vi "Convert Write ERD List to Message.vi"(0 "GEA Inputs":T1 {"Destination" format="%.0x"; "Source" format="%.0x"}, 7 "Write ERD List":T3[](array[typedef]) {"ERD Number" format="%.0x"}, 11 "Error In":errorcluster) -> (4 "GEA Message":T2 {"Command" format="%02x"; "Destination" format="%02x"; "Source" format="%02x"}, 15 "Error Out":errorcluster)   [LabVIEW 2016, in "GEA2_Toolkit.lvlib"]
doc: "This vi uses the Source / Destination from the GEA input and the ERD Write list to format a single GEA2 message to read the list of ERDs."
uses:
  library/GEA2_Toolkit.lvlib
  type defs/ERD Write Data In.ctl
  type defs/Data Type.ctl
  type defs/Data In.ctl
  type defs/Source_Destination.ctl
  <vilib>/regexp/Match Regular Expression.xnode
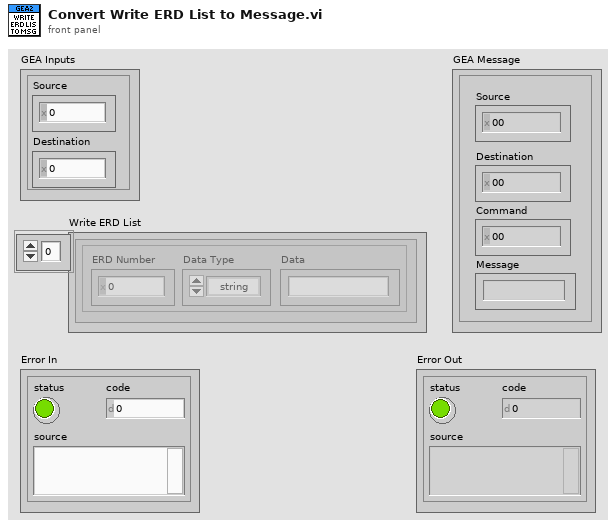
[diagram p1: front panel]
types:
  T1 = typedef "GEA2_Toolkit.lvlib/Source_Destination.ctl" = cluster{"Source":u8, "Destination":u8}
  T2 = typedef "GEA2_Toolkit.lvlib/Data In.ctl" = cluster{"Source":u8, "Destination":u8, "Command":u8, "Message":string}
  T3 = typedef "GEA2_Toolkit.lvlib/ERD Write Data In.ctl" = cluster{"ERD Number":u16, "Data Type":T4, "Data":string}
  T4 = typedef "GEA2_Toolkit.lvlib/Data Type.ctl" = enum16{"string", "boolean", "uint8_t", "uint16_t", "uint32_t", "uint64_t"}
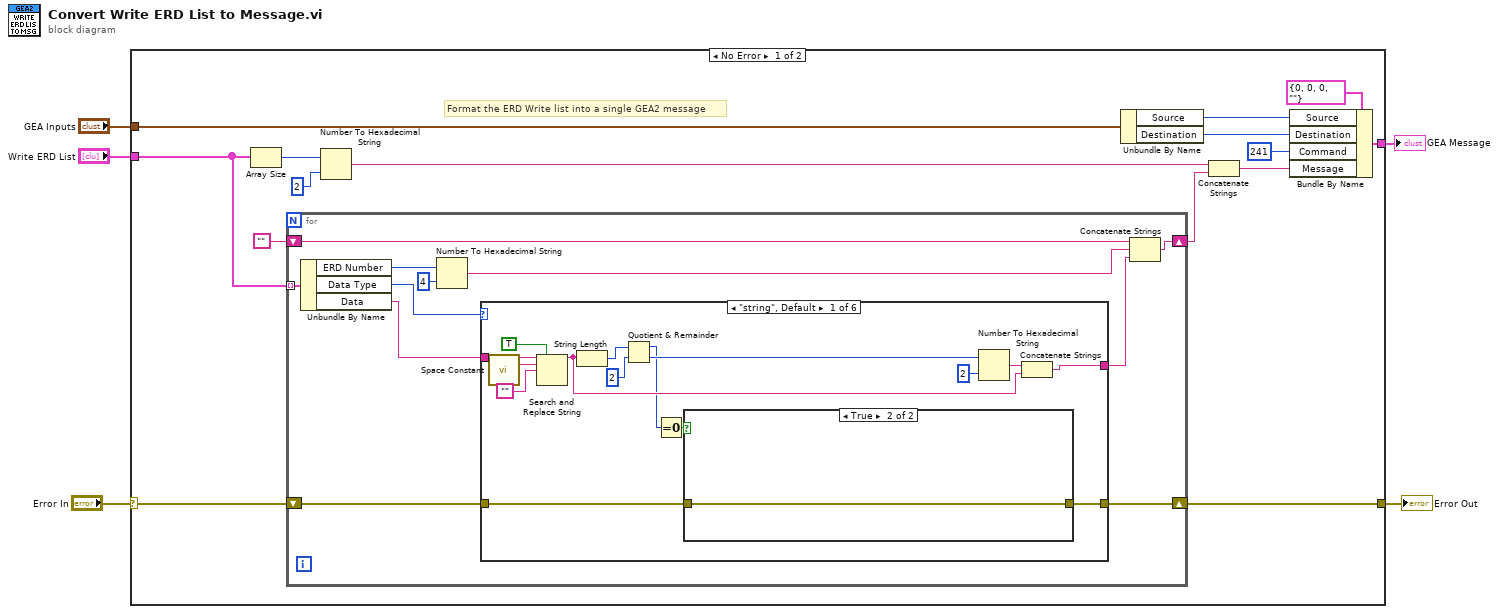
[diagram p0: block diagram]
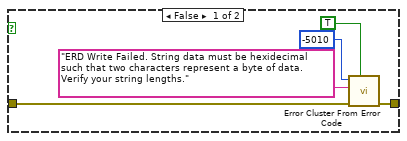
[diagram p2: hidden frame]
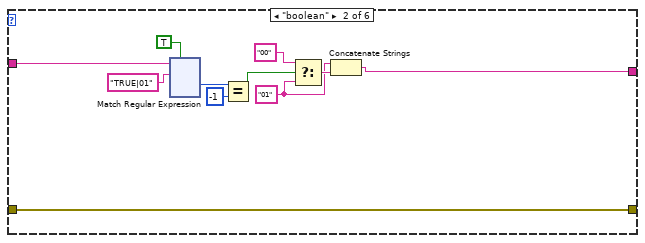
[diagram p3: hidden frame]
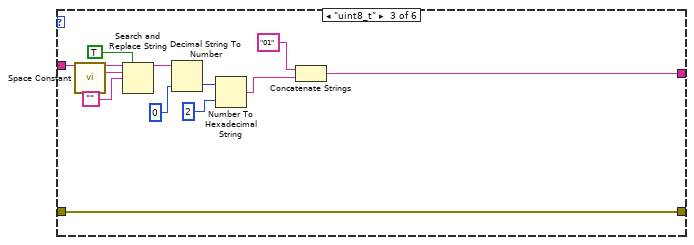
[diagram p4: hidden frame]
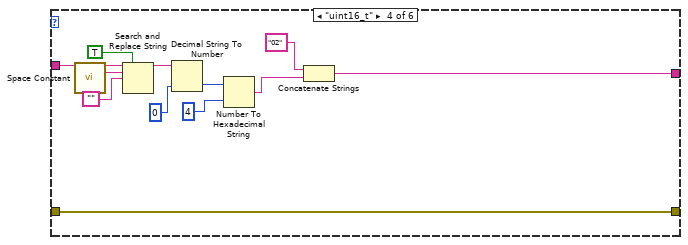
[diagram p5: hidden frame]
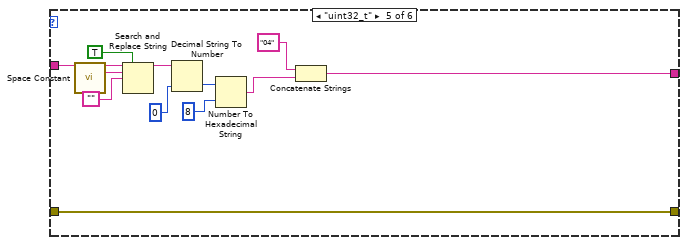
[diagram p6: hidden frame]
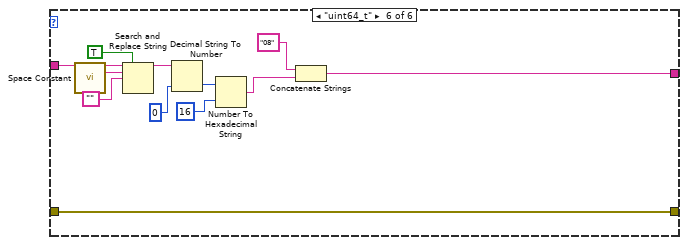
[diagram p7: hidden frame]
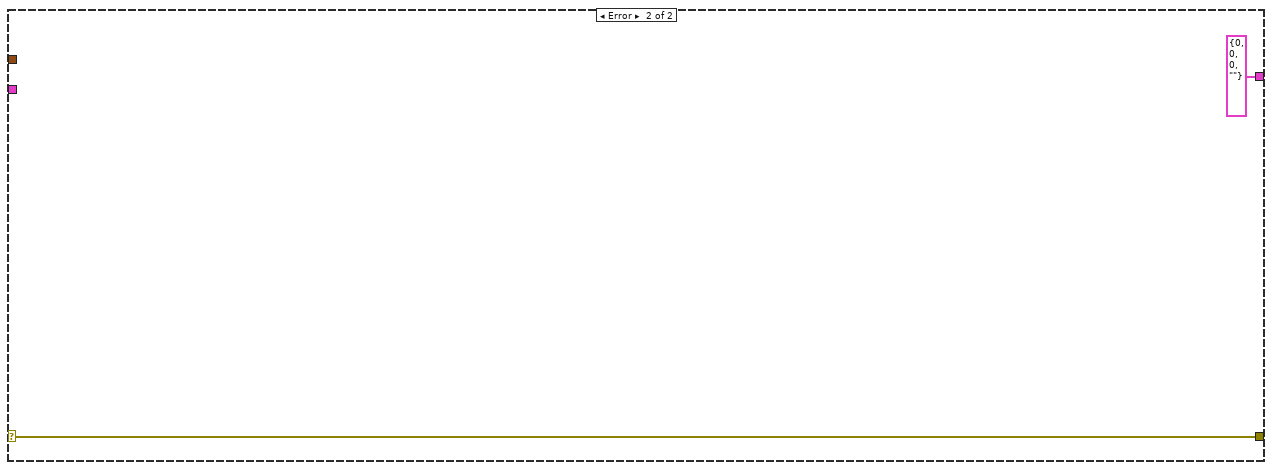
[diagram p8: hidden frame]
diagram:
  n1 = case shown="No Error" "Error In" {
    selector: "Error In" -> [w7 w227]
    tunnel: "Write ERD List" -> [w17 _]
    tunnel: "GEA Inputs" -> [w13 _]
    tunnel: [w8 T2 {"Source"=0, "Destination"=0, "Command"=0, "Message"=""} ("GEA Message")] -> w3
    tunnel: [w6 w227] -> w1
    frame No Error {
      # "Format the ERD Write list into a single GEA2 message"
      n2 = Array Size(array=w17) -> (size(s)=w19:i32)
      n3 = for {
        tunnel: w17 -> [w31] mode=indexing
        shift-right: [w26] -> w15
        shift-left: "" -> [w28]
        shift-right: [w21] -> w6
        shift-left: w7 -> [w22]
        n4 = Unbundle By Name(w31) -> ("ERD Number"=w30:u16, "Data Type"=w25:T4, "Data"=w24:string)
        n5 = Number To Hexadecimal String(1:i16 4 ("width (-)"), 2:w30) -> (0:w27:string)
        n6 = case shown="\"string\", Default" w25 {
          tunnel: w24 -> [w46 w62 w186 w193 w205 w217]
          tunnel: [w41 w55 w185 w194 w204 w216] -> w23
          tunnel: w22 -> [w35 w53 w178 w192 w203 w215]
          tunnel: [w32 w53 w178 w192 w203 w215] -> w21
          frame "string", Default {
            n7 = call <vilib>:"Space Constant.vi"() -> ("String"=w44:string)
            n8 = Search and Replace String(replace all?=TRUE ("replace all? (F)"), input string=w46, search string=w44, replace string="") -> (result string=w40:string)  [unwired: 4 in, 3 out]
            n9 = String Length(string=w40) -> (length=w38:i32)
            n10 = Quotient & Remainder(x=w38, y=2) -> (x-y*floor(x/y)=w34:i32, floor(x/y)=w37:i32)
            n11 = Equal To 0?(x=w34) -> (x = 0?=w33:bool)
            n12 = case shown="True" w33 {
              tunnel: w35 -> [w51 w52]
              tunnel: [w47 w52] -> w32
              frame False {
                n13 = call <vilib>:"Error Cluster From Error Code.vi"("show call chain? (False)"=TRUE, "error in (no error)"=w51, "error message (\"\")"="ERD Write Failed. String data must be hexidecimal such that two characters represent a byte of data. Verify your string lengths." ("error message (\"\")"), "error code (0)"=-5010) -> ("error out"=w47:errorcluster)  [unwired: 5 in]
              }
              frame True {
              }
            }
            n14 = Number To Hexadecimal String(1:i16 2 ("width (-)"), 2:w37) -> (0:w42:string)
            n15 = Concatenate Strings(w42, w40) -> (w41:string)
          }
          frame "boolean" {
            w54 = "01"
            n16 = xnode "Match Regular Expression"("input string"=w62, "regular expression"="TRUE|01", "ignore case? (F)"=TRUE) -> ("offset past match"=w60:i32)  [unwired: 3 in, 4 out]
            n17 = Equal?(x=w60, y=-1) -> (x = y?=w57:bool)
            n18 = Select(t="00", s=w57, f=w54) -> (s? t:f=w56:string)
            n19 = Concatenate Strings(w54, w56) -> (w55:string)
          }
          frame "uint8_t" {
            n20 = call <vilib>:"Space Constant.vi"() -> ("String"=w188:string)
            n21 = Search and Replace String(replace all?=TRUE ("replace all? (F)"), input string=w186, search string=w188, replace string="") -> (result string=w183:string)  [unwired: 4 in, 3 out]
            n22 = Decimal String To Number(string=w183, default (0L)=u8 0) -> (number=w180:u8)  [unwired: 1 in, 1 out]
            n23 = Number To Hexadecimal String(1:i16 2 ("width (-)"), 2:w180) -> (0:w179:string)
            n24 = Concatenate Strings("01", w179) -> (w185:string)
          }
          frame "uint16_t" {
            n25 = call <vilib>:"Space Constant.vi"() -> ("String"=w200:string)
            n26 = Search and Replace String(replace all?=TRUE ("replace all? (F)"), input string=w193, search string=w200, replace string="") -> (result string=w190:string)  [unwired: 4 in, 3 out]
            n27 = Decimal String To Number(string=w190, default (0L)=u16 0) -> (number=w195:u16)  [unwired: 1 in, 1 out]
            n28 = Number To Hexadecimal String(1:i16 4 ("width (-)"), 2:w195) -> (0:w191:string)
            n29 = Concatenate Strings("02", w191) -> (w194:string)
          }
          frame "uint32_t" {
            n30 = call <vilib>:"Space Constant.vi"() -> ("String"=w212:string)
            n31 = Search and Replace String(replace all?=TRUE ("replace all? (F)"), input string=w205, search string=w212, replace string="") -> (result string=w209:string)  [unwired: 4 in, 3 out]
            n32 = Decimal String To Number(string=w209, default (0L)=u32 0) -> (number=w206:u32)  [unwired: 1 in, 1 out]
            n33 = Number To Hexadecimal String(1:i16 8 ("width (-)"), 2:w206) -> (0:w202:string)
            n34 = Concatenate Strings("04", w202) -> (w204:string)
          }
          frame "uint64_t" {
            n35 = call <vilib>:"Space Constant.vi"() -> ("String"=w224:string)
            n36 = Search and Replace String(replace all?=TRUE ("replace all? (F)"), input string=w217, search string=w224, replace string="") -> (result string=w221:string)  [unwired: 4 in, 3 out]
            n37 = Decimal String To Number(string=w221, default (0L)=u32 0) -> (number=w218:u32)  [unwired: 1 in, 1 out]
            n38 = Number To Hexadecimal String(1:i16 16 ("width (-)"), 2:w218) -> (0:w214:string)
            n39 = Concatenate Strings("08", w214) -> (w216:string)
          }
        }
        n40 = Concatenate Strings(w28, w27, w23) -> (w26:string)
      }
      n41 = Number To Hexadecimal String(1:i16 2 ("width (-)"), 2:w19) -> (0:w18:string)
      n42 = Unbundle By Name(w13) -> ("Source"=w12:u8, "Destination"=w11:u8)
      n43 = Concatenate Strings(w18, w15) -> (w9:string)
      n44 = Bundle By Name(cluster=T2 {"Source"=0, "Destination"=0, "Command"=0, "Message"=""} ("GEA Message"), "Source"=w12, "Destination"=w11, "Command"=u8 241, "Message"=w9) -> (w8:T2)
    }
    frame Error {
    }
  }
  "GEA Message" <- w3
  "Error Out" <- w1
